vi "Audio Plugin UI Meas Ser1.vi"() -> ()   [LabVIEW 2021]
uses:
  <vilib>/PDM Acquisition Toolkit/shared/controls/i2s frame size.ctl
  <vilib>/PDM Acquisition Toolkit/host/Classes/Tasks/PDM Tasks/Controls/Acquisition Mode.ctl
  <vilib>/addons/_NISVFA/_Shared subVIs/Controls/svc_Window.ctl
  <vilib>/addons/_NISVFA/_Shared subVIs/Common/SVL Set dB Reference (1 Ch).vi
  <vilib>/addons/Sound and Vibration/svt_Level/SVL AC & DC Level (Time) (1 Ch).vi
  <vilib>/addons/_NISVFA/_Spectrum Processing/SVFA Get Spectrum Subset.vi
  <vilib>/addons/_NISVFA/_Spectrum Processing/SVFA Get Spectrum Subset (Complex) (1 Ch).vi
  <vilib>/addons/_NISVFA/_Shared subVIs/Common/svc_Window Parameters.vi
  <vilib>/addons/_NISVFA/_Shared subVIs/Common/svc_Extract Single Tone Information (complex).vi
  <vilib>/addons/_NISVFA/_Shared subVIs/Common/svc_Check Frequency Range in Spectrum.vi
  <vilib>/addons/_NISVFA/_Spectrum Processing/SVFA Unit Conversion.vi
  <vilib>/addons/_NISVFA/_Spectrum Processing/SVFA Unit Conversion (Complex) (1 Ch).vi
  <vilib>/addons/_NISVFA/_Spectrum Processing/SVFA Spectrum Peak Search.vi
  <vilib>/addons/_NISVFA/_Spectrum Processing/SVFA Spectrum Peak Search (1 Ch).vi
  <vilib>/addons/_NISVFA/_Shared subVIs/Common/svc_Spectrum Units.vi
  <vilib>/addons/_NISVFA/_Shared subVIs/Common/SVL Set dB Reference (variant).vi
  <vilib>/addons/_NISVFA/_Shared subVIs/Common/svc_Get SV Channel Info.vi
  <vilib>/Analysis/baseanly.llb/Mean.vi
  <vilib>/Analysis/baseanly.llb/Mean (DBL).vi
  <vilib>/addons/_NISVFA/_Shared subVIs/Windowing/svfa_Scaled Time Domain Window (Array).vi
  <vilib>/addons/_NISVFA/_Shared subVIs/Common/svc_Build Unit Label for Frequency Range.vi
  <vilib>/addons/_NISVFA/_Spectrum Processing/SVFA Get Tone Amplitude and Phase (1 Ch).vi
  <vilib>/addons/_NISVFA/_Spectrum Processing/subVIs/svfa_Compute Complex Spectrum for Export.vi
  <vilib>/addons/_NISVFA/_Shared subVIs/Common/svc_Check Frequency Range in Bandwidth.vi
  <vilib>/addons/_NISVFA/_Shared subVIs/Common/svc_Convert Start and Stop to Start Index and Length.vi
  <vilib>/addons/_NISVFA/_Shared subVIs/Common/svc_Log View for Spectrum (1Ch).vi
  <vilib>/addons/_NISVFA/_Spectrum Processing/SVFA Unit Conversion (1 Ch).vi
  <vilib>/addons/_NISVFA/_Shared subVIs/Common/svc_Complex Datatype Defaults.vi
  <vilib>/addons/_NISVFA/_Spectrum Processing/subVIs/svfa_Spectrum Peak Search.vi
  <vilib>/addons/_NISVFA/_Shared subVIs/Common/svc_Format Value (DBL).vi
  <vilib>/addons/_NISVFA/_Shared subVIs/Common/svc_Get Weighting Enum and Labels.vi
  <vilib>/addons/_NISVFA/_Shared subVIs/Common/svc_Engineering Units to Unit Label.vi
  <vilib>/addons/_NISVFA/_Shared subVIs/Common/svc_Surround NonAlpha String with Parentheses.vi
  <vilib>/dlg_ctls.llb/Space Constant.vi
  <vilib>/addons/_NISVFA/_Shared subVIs/Common/svc_Unit Label to Engineering Units.vi
  <vilib>/addons/_NISVFA/_Spectrum Processing/subVIs/svfa_Spectrum Info Window to windowTd Type Def.vi
  <vilib>/Analysis/4window.llb/Force Window.vi
  <vilib>/Analysis/4window.llb/Force Window (DBL).vi
  <vilib>/Analysis/4window.llb/Exponential Window.vi
  <vilib>/Analysis/4window.llb/Exponential Window (DBL).vi
  <vilib>/addons/_NISVFA/_Spectrum Processing/subVIs/svfa_Window Frequency Response.vi
  <vilib>/addons/_NISVFA/_Spectrum Processing/subVIs/svfa_Window Frequency Response (double array).vi
  <vilib>/Analysis/baseanly.llb/Dot Product.vi
  <vilib>/Analysis/baseanly.llb/Complex Dot Product.vi
  <vilib>/addons/_NISVFA/_Shared subVIs/Common/svc_Unwrap Phase.vi
  <vilib>/addons/_NISVFA/_Shared subVIs/Common/svc_Convert Spectrum Array to dB.vi
  <vilib>/addons/_NISVFA/_Spectrum Processing/subVIs/svfa_Conversion Utility (spectrum info).vi
  <vilib>/addons/_NISVFA/_Spectrum Processing/subVIs/svfa_Peak Rough Search Indices.vi
  <vilib>/addons/_NISVFA/_Shared subVIs/Common/svc_Unit Label Lexical Class.vi
  <vilib>/addons/_NISVFA/_Spectrum Processing/subVIs/svfa_Rect Window Frequency Response.vi
  <vilib>/addons/_NISVFA/_Spectrum Processing/subVIs/svfa_Cosine Window Coefficients.vi
  <vilib>/addons/_NISVFA/_Spectrum Processing/subVIs/svfa_Peak to RMS to Peak2Peak.vi
  <vilib>/addons/_NISVFA/_Spectrum Processing/subVIs/svfa_Mag to Mag2.vi
  <vilib>/addons/_NISVFA/_Spectrum Processing/subVIs/svfa_Linear to dB.vi
  <vilib>/addons/_NISVFA/_Spectrum Processing/subVIs/svfa_dBrefA to dBrefB.vi
  <vilib>/addons/_NISVFA/_Spectrum Processing/subVIs/svfa_Spectrum to Spectral Density.vi
  <vilib>/PDM Acquisition Toolkit/host/API/Public/Create Tasks/Create I2S Input Task.vi
  <vilib>/PDM Acquisition Toolkit/host/API/Public/Configure/Timing/Configure Timing - I2S Input Slave.vi
  <vilib>/PDM Acquisition Toolkit/host/API/Public/Configure/PDM Channel/Configure Microphone Sensitivity FSPA - I2S Input Task.vi
  <vilib>/PDM Acquisition Toolkit/host/API/Public/Commit/Commit I2S Input Task.vi
  <vilib>/DAQmx/create/channels.llb/DAQmx Create Channel (AO-FuncGen).vi
  <vilib>/addons/_NISVFA/_Shared subVIs/Common/svc_Caller VI Returned in Error Source.vi
  <vilib>/addons/_NISVFA/_Shared subVIs/Common/svc_Get Window Info.vi
  <vilib>/Analysis/0measdsp.llb/Scaled Time Domain Window.vi
  <vilib>/Analysis/0measdsp.llb/Scaled Time Domain Window (DBL).vi
  <vilib>/Utility/error.llb/Error Cluster From Error Code.vi
  <vilib>/Analysis/baseanly.llb/Std Deviation and Variance.vi
  <vilib>/addons/Sound and Vibration/svt_Distortion/subVIs/sv_Check Data Valid (Audio) (1 Ch).vi
  <vilib>/addons/_NISVFA/_Shared subVIs/Common/svc_Convert Frequency to Frequency String.vi
  <vilib>/Analysis/4window.llb/window parameters.vi
  <vilib>/Analysis/4window.llb/Window Properties.vi
  <vilib>/Analysis/4window.llb/Window Properties by Name.vi
  <vilib>/addons/_NISVFA/_Spectrum Processing/subVIs/svfa_Spectrum Peak Tone Search and Estimation (complex).vi
  <vilib>/measure/masignal.llb/Tones and Noise Waveform.vi
  <vilib>/addons/_NISVFA/_Shared subVIs/Common/svc_FFT with Window.vi
  <vilib>/Analysis/1siggen.llb/Square Wave.vi
  <vilib>/addons/_NISVFA/_Spectrum Processing/subVIs/svfa_Three Finger Peak Search.vi
  <vilib>/addons/Sound and Vibration/svt_Distortion/subVIs/sv_Peak View Amplitude (1 Ch).vi
  <vilib>/addons/Sound and Vibration/svt_Level/SVL AC & DC Level (Time) (N Ch).vi
  <vilib>/addons/_NISVFA/_Shared subVIs/Common/SVL Set dB Reference (N Ch - 1 Ref).vi
  <vilib>/addons/Sound and Vibration/svt_Single Tone Measurements/SVT Dynamic Range (Frequency) (1 Ch).vi
  <vilib>/addons/Sound and Vibration/svt_Distortion/SVT SNR without Harmonics (Frequency) (1 Ch).vi
  <vilib>/addons/Sound and Vibration/svt_Single Tone Measurements/SVT Gain (Time) (1 Ch).vi
  <vilib>/PDM Acquisition Toolkit/host/API/Public/Start/Start I2S Input Task.vi
  <vilib>/PDM Acquisition Toolkit/host/API/Public/Read/Read I2S Waveform.vi
  <vilib>/PDM Acquisition Toolkit/host/API/Public/Clear/Clear I2S Input Task.vi
  <vilib>/addons/Sound and Vibration/svt_Single Tone Measurements/SVT Spurious Free Dynamic Range (Frequency) (1 Ch).vi
  <vilib>/addons/Sound and Vibration/svt_Weighting/SVT Weighting Filter (N Ch).vi
  <vilib>/PDM Acquisition Toolkit/host/Classes/Tasks/PDM Tasks/PDM Task.lvclass
  <vilib>/PDM Acquisition Toolkit/host/API/PDM Acquisition Toolkit.lvlib
  <vilib>/addons/Sound and Vibration/svt_Single Tone Measurements/SoundVib_SingleTone.lvlib
  <vilib>/addons/Sound and Vibration/svt_Distortion/SoundVib_Distortion.lvlib
  <vilib>/PDM Acquisition Toolkit/shared/PDM Shared.lvlib
  <vilib>/addons/Sound and Vibration/svt_Weighting/SoundVib_ABCWeighting.lvlib
panel:
  out "MeasTable":string[][](table)
  out "MeasGraphs":enum32{"Time Domain", "Histogram", "DNL", "INL"}(tab)
  out "TimeDomain":waveform(dbl)[](graph) caption="AC"
  in  "Weighting":T1(ring) caption="WEIGHTING"
  in  "Bits per Sample":u32=24 caption="BITS PER SAMPLE"
  in  "DUT FULL SCALE (V pk)":dbl=3.16 format="%.3p"
  out "error out":errorcluster
  out "Sampling Rate":dbl=192000.0 format="%#_6p"
  in  "sample rate (S/s)":dbl=192000.0
  in  "Playback .WAV File?":bool caption="PLAYBACK .WAV FILE?"
  in  "I2S Data Latch at SCK Cycle":u8=50 caption="DATA LATCH AT SCK" format="%.0f%"
  in  "I2S Logic Level":enum16{"3.3 V", "1.8 V", "1.2 V"}(ring) caption="LOGIC LEVEL"
  in  "I2S Frame Size":enum16{"32bits", "64bits"}(ring) caption="FRAME SIZE"
  in  "I2S Number of Words":u32=19200 caption="NO OF WORDS"
  in  "I2S Word Length":u32=24 caption="WORD LENGTH"
  in  "I2S Clock Rate":u32=12288000 caption="CLOCK RATE" format="%#.6pHz"
  in  "THD Maximum Harmonic":u32=9 caption="MAX HARMONIC"
  in  "Measurement Band Stop":dbl=20000.0 caption="BAND STOP" format="%#_6pHz"
  in  "Measurement Band Start":dbl=20.0 caption="BAND START" format="%#_6pHz"
  in  "DSG amplitude":dbl=1.0 caption="AMPLITUDE" format="%#_6pV"
  in  "DSG frequency":dbl=1000.0 caption="FREQUENCY" format="%#_6pHz"
  in  "DSG resource name":string="4468/ao0" caption="RESOURCE NAME"
  in  "Mic sensitivity (FS/Pa)":dbl=0.34762 caption="MIC SENSITIVITY" format="%.3fFS/Pa"
  in  "I2S Channel List":string="PXI1Slot7\\I2Si 0" caption="CHANNEL LIST"
  in  "Playback .WAV file path":path caption="PLAYBACK .WAV FILE PATH"
  in  "Record .WAV File?":bool caption="RECORD .WAV FILE?"
  in  "Record wave file path":path caption="RECORD .WAV FILE PATH"
  # "Analog Source"
  # "I2S Setting"
  # "Measurement"
  # "Record"
  # "Playback"
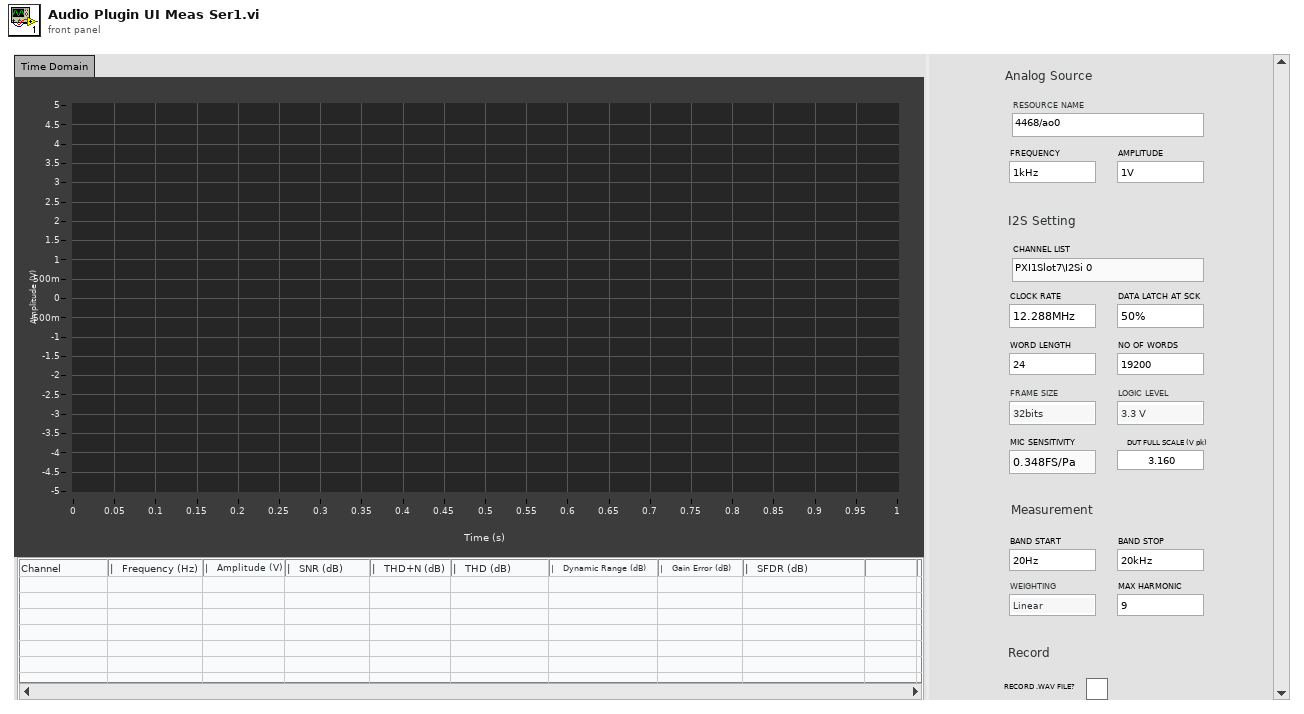
[diagram p1: front panel]
types:
  T1 = enum16{"Linear", "A-Weighting", "B-Weighting", "C-Weighting"}
  T2 = cluster{"band start (Hz)":dbl, "band stop (Hz)":dbl}
  T3 = typedef "PDM Shared.lvlib/i2s frame size.ctl" = enum16{"32bits", "64bits"}
  T4 = cluster{"frequency range":cluster{"band start (Hz)":dbl, "band stop (Hz)":dbl}, "THD maximum harmonic":i32, "amplitude":dbl, "frequency (Hz)":dbl, "output channel":tag, "microphone sensitivity (FS/Pa)":dbl, "number of words":i32, "channel list":string, "logic level":enum16{"3.3 V", "1.8 V", "1.2 V"}, "I2S serial clock rate 2":u32, "frame size":T3, "word length":u32, "Data Latch at SCK cycle":u8, "Playback .WAV File?":bool, "Record .WAV File?":bool, "Record wave file path":path, "Playback .WAV file path":path, "number of channels":i32, "DUT full scale (V pk)":dbl, "weighting":u16}
  T5 = typedef "PDM Acquisition Class Library.lvlib/PDM Task.lvclass/Acquisition Mode.ctl" = enum16{"Finite", "Continuous"}
  T6 = cluster{"SNR units":enum16{"dB", "linear ratio", "%"}, "detected fundamental amplitude units":enum16{"EU rms", "EU peak", "EU peak-peak"}}
  T7 = cluster{"gain units":enum16{"dB", "linear ratio"}, "detected fundamental amplitude units":enum16{"EU rms", "EU peak", "EU peak-peak"}}
  T8 = typedef "PDM Acquisition Class Library.lvlib/I2S Input Task.lvclass/DVR I2S Input Task.ctl" = refnum<data-value>
  T9 = typedef "svc_Window.ctl" = u32
  T10 = typedef "svc_Spectrum Info.ctl" = cluster{"channel name":string, "description":string, "x-axis units":T11, "spectral info":cluster{"spectrum type":T12, "linear/dB":enum16{"linear", "dB"}, "window":u16, "window size":i32, "FFT size":i32}, "engineering units":T13, "custom label":string, "dB reference [EU]":dbl, "peak units":enum16{"rms", "peak", "peak-peak"}, "weighting filter":T14, "spectral density?":bool, "unit label":string, "spectrum skewed?":bool, "complimentary spectrum units":T15}
  T11 = typedef "svc_X-Axis Units.ctl" = u16
  T12 = typedef "svc_Spectrum Type.ctl" = enum16{"FFT Spectrum [complex]", "Amplitude [Magnitude]", "Power [Magnitude^2]", "Cross Spectrum [complex]", "Frequency Response [Complex]"}
  T13 = typedef "svc_Engineering Units Text Ring.ctl" = u16
  T14 = typedef "svc_Weighting Filter Text Ring.ctl" = u16
  T15 = typedef "svc_Complimentary Spectrum Units.ctl" = enum16{"none", "radians", "degrees", "cycles", "imaginary"}
  T16 = cluster{"complex spectrum response":cluster{"f0":dbl, "df":dbl, "complex spectrum":cdb[]}, "spectrum info":T10}
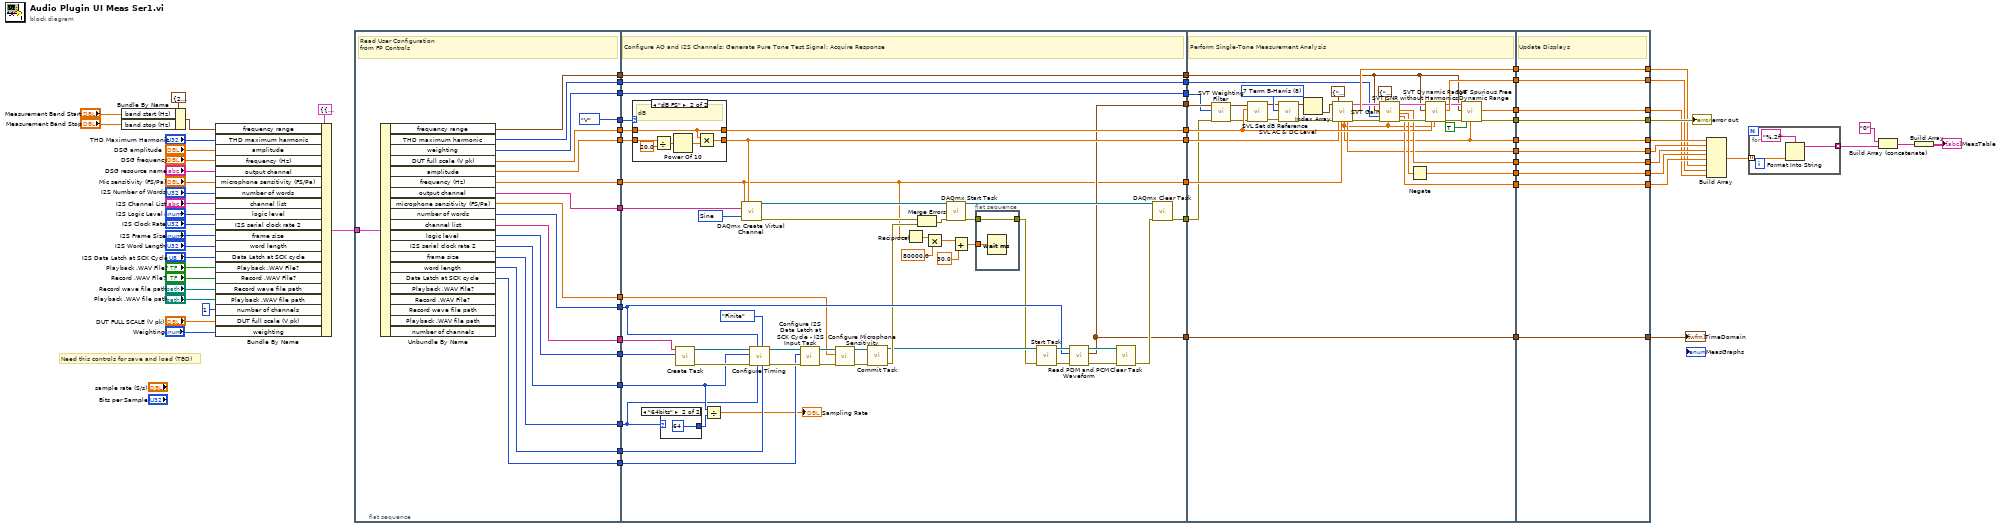
[diagram p0: block diagram]
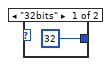
[diagram p2: hidden frame]
diagram:
  # "Need this controls for save and load (TBD)"
  n1 = Bundle By Name(cluster=T2 {"band start (Hz)"=20.0, "band stop (Hz)"=20000.0} ("frequency range"), "band start (Hz)"="Measurement Band Start", "band stop (Hz)"="Measurement Band Stop") -> (w41:T2)
  n2 = Bundle By Name(cluster=T4 {"frequency range"={"band start (Hz)"=20.0, "band stop (Hz)"=20000.0}, "THD maximum harmonic"=9, "amplitude"=1.0, "frequency (Hz)"=1000.0, "output channel"="Dev1/ao0", "microphone sensitivity (FS/Pa)"=0.34762, "number of words"=19200, "channel list"="PXI1Slot7\\I2Si 0", "logic level"=enum."3.3 V", "I2S serial clock rate 2"=12288000, "frame size"=enum."64bits", "word length"=24, "Data Latch at SCK cycle"=50, "Playback .WAV File?"=FALSE, "Record .WAV File?"=FALSE, "Record wave file path"=path "", "Playback .WAV file path"=path "", "number of channels"=1, "DUT full scale (V pk)"=3.16, "weighting"=0}, "frequency range"=w41, "THD maximum harmonic"="THD Maximum Harmonic", "amplitude"="DSG amplitude", "frequency (Hz)"="DSG frequency", "output channel"="DSG resource name", "microphone sensitivity (FS/Pa)"="Mic sensitivity (FS/Pa)", "number of words"="I2S Number of Words", "channel list"="I2S Channel List", "logic level"="I2S Logic Level", "I2S serial clock rate 2"="I2S Clock Rate", "frame size"="I2S Frame Size", "word length"="I2S Word Length", "Data Latch at SCK cycle"="I2S Data Latch at SCK Cycle", "Playback .WAV File?"="Playback .WAV File?", "Record .WAV File?"="Record .WAV File?", "Record wave file path"="Record wave file path", "Playback .WAV file path"="Playback .WAV file path", "number of channels"=1, "DUT full scale (V pk)"="DUT FULL SCALE (V pk)", "weighting"="Weighting") -> (w23:T4)
  n3 = flat-sequence {
    tunnel: [w89] -> w75
    tunnel: [w86] -> w74
    tunnel: [w85] -> w73
    tunnel: [w88] -> w72
    tunnel: [w87] -> w71
    tunnel: [enum16{"V", "dB FS"}."V" ("amplitude units")] -> w70
    tunnel: [w80] -> w69
    tunnel: [w81] -> w68
    tunnel: [w77] -> w67
    tunnel: [w83] -> w66
    tunnel: [w78] -> w65
    tunnel: [w79] -> w64
    tunnel: [w82] -> w63
    tunnel: [w84] -> w47
    tunnel: w23 -> [w91]
    tunnel: [w90] -> w22
    tunnel: [w76] -> w3
    tunnel: w75 -> [w138]
    tunnel: w74 -> [w98]
    tunnel: w73 -> [w136]
    tunnel: w72 -> [w141]
    tunnel: w71 -> [w140]
    tunnel: w70 -> [w137]
    tunnel: [w142] -> w62
    tunnel: [w139] -> w61
    tunnel: [w138] -> w60
    tunnel: [w135] -> w59
    tunnel: [w98] -> w58
    tunnel: [w106] -> w57
    tunnel: [w130] -> w56
    tunnel: w69 -> [w117]
    tunnel: w68 -> [w116]
    tunnel: w67 -> [w115]
    tunnel: w66 -> [w114]
    tunnel: w65 -> [w113]
    tunnel: w64 -> [w112]
    tunnel: w63 -> [w111]
    tunnel: w47 -> [w108]
    tunnel: w22 -> [w142]
    tunnel: [w106] -> w18
    tunnel: w3 -> [w105]
    tunnel: [w105] -> w2
    tunnel: [w178] -> w55
    tunnel: [w177] -> w54
    tunnel: [w164] -> w53
    tunnel: [w176] -> w52
    tunnel: [w175] -> w51
    tunnel: [w174] -> w50
    tunnel: [w173] -> w49
    tunnel: [w163] -> w48
    tunnel: w62 -> [w162]
    tunnel: w61 -> [w180]
    tunnel: w60 -> [w170]
    tunnel: w59 -> [w179]
    tunnel: w58 -> [w172]
    tunnel: w57 -> [w159]
    tunnel: w56 -> [w156]
    tunnel: [w167] -> w19
    tunnel: w18 -> [w167]
    tunnel: [w160] -> w17
    tunnel: w2 -> [w155]
    tunnel: w55 -> [w193]
    tunnel: w54 -> [w192]
    tunnel: w53 -> [w200]
    tunnel: w52 -> [w194]
    tunnel: w51 -> [w195]
    tunnel: w50 -> [w196]
    tunnel: w49 -> [w197]
    tunnel: w48 -> [w198]
    tunnel: [w200] -> w46
    tunnel: [w199] -> w20
    tunnel: w19 -> [w199]
    tunnel: w17 -> [w191]
    tunnel: [w198] -> w16
    tunnel: [w197] -> w15
    tunnel: [w196] -> w14
    tunnel: [w195] -> w13
    tunnel: [w194] -> w12
    tunnel: [w193] -> w11
    tunnel: [w192] -> w10
    tunnel: [w191] -> w9
    frame #0 {
      # "Read User Configuration\nfrom FP Controls"
      n4 = Unbundle By Name(w91) -> ("frequency range"=w90:T2, "THD maximum harmonic"=w89:i32, "weighting"=w76:u16, "DUT full scale (V pk)"=w88:dbl, "amplitude"=w87:dbl, "frequency (Hz)"=w86:dbl, "output channel"=w85:tag, "microphone sensitivity (FS/Pa)"=w84:dbl, "number of words"=w83:i32, "channel list"=w82:string, "logic level"=w81:enum16{"3.3 V", "1.8 V", "1.2 V"}, "I2S serial clock rate 2"=w80:u32, "frame size"=w79:T3, "word length"=w78:u32, "Data Latch at SCK cycle"=w77:u8)  [unwired: 5 out]
    }
    frame #1 {
      w107 = 14751 items=["Sine"=14751, "Triangle"=14752, "Square"=14753, "Sawtooth"=14754] ("type")
      # "Configure AO and I2S Channels; Generate Pure Tone Test Signal; Acquire Response"
      n5 = case shown="\"dB FS\"" w137 {
        tunnel: [w148 w150] -> w135
        tunnel: w140 -> [w148 w154]
        tunnel: w141 -> [w147 w149]
        tunnel: [w147 w149] -> w139
        frame Default {
          # "V"
        }
        frame "dB FS" {
          # "dB"
          n6 = Divide(x=w154, y=20.0) -> (x/y=w152:dbl)
          n7 = Power Of 10(x=w152) -> (10^x=w151:dbl)
          n8 = Multiply(x=w149, y=w151) -> (x*y=w150:dbl)
        }
      }
      n9 = case shown="\"64bits\"" w112 {
        tunnel: [u8 32 ("frame size") u8 64 ("frame size")] -> w118
        frame "32bits" {
        }
        frame "64bits" {
        }
      }
      n10 = call-poly <vilib>:"Create Task.vi"("logic level"=w116, "channel list"=w111) -> ("error out"=w124:errorcluster, "I2S input task out"=w123:T8)  [unwired: 8 in]
      n11 = Divide(x=w117, y=w118) -> (x/y=→"Sampling Rate":dbl)
      n12 = call-poly <vilib>:"DAQmx Create Virtual Channel.vi"("frequency"=w98, "amplitude"=w135, "physical channels"=w136, "type"=w107) -> ("task out"=w132:refnum<k21>, "error out"=w134:errorcluster)  [unwired: 10 in]
      n13 = call-poly <vilib>:"Configure Timing.vi"("word length"=w113, "acquisition mode"=Acquisition_Mode."Finite", "frame size"=w112, "number of words"=w114, "error in"=w124, "I2S serial clock rate"=w117, "I2S input task in"=w123) -> ("error out"=w122:errorcluster, "I2S input task out"=w119:T8)  [unwired: 3 in]
      n14 = call <vilib>:"Configure I2S Data Latch at SCK Cycle - I2S Input Task.vi"("error in"=w122, "data latch at SCK cycle"=w115, "I2S input task in"=w119) -> ("error out"=w121:errorcluster, "I2S input task out"=w120:T8)  [unwired: 7 in]
      n15 = call-poly <vilib>:"Configure Microphone Sensitivity.vi"("error in"=w121, "microphone sensitivity (FS/Pa)"=w108, "I2S input task in"=w120) -> ("error out"=w104:errorcluster, "I2S input task out"=w103:T8)  [unwired: 7 in]
      n16 = call-poly <vilib>:"Commit Task.vi"("error in"=w104, "I2S input task in"=w103) -> ("error out"=w102:errorcluster, "I2S input task out"=w101:T8)  [unwired: 8 in]
      n17 = Reciprocal(x=w98) -> (1/x=w97:dbl)
      n18 = Merge Errors(w134, w102) -> (w133:errorcluster)
      n19 = Multiply(x=w97, y=80000.0) -> (x*y=w95:dbl)
      n20 = call <vilib>:"DAQmx Start Task.vi"("task/channels in"=w132, "error in"=w133) -> ("task out"=w131:refnum<k21>, "error out"=w99:errorcluster)  [unwired: 12 in]
      n21 = Add(x=w95, y=30.0) -> (x+y=w93:dbl)
      n22 = flat-sequence {
        tunnel: [w144] -> w100
        tunnel: w99 -> [w144]
        tunnel: w93 -> [w143]
        frame #0 {
          n23 = Wait (ms)(milliseconds to wait=w143) -> ()  [unwired: 1 out]
        }
      }
      n24 = call-poly <vilib>:"Start Task.vi"("error in"=w100, "I2S input task in"=w101) -> ("error out"=w128:errorcluster, "I2S input task out"=w127:T8)  [unwired: 8 in]
      n25 = call-poly <vilib>:"Read PDM and PCM Waveform.vi"("error in"=w128, "words per channel"=w114, "I2S input task in"=w127) -> ("error out"=w126:errorcluster, "I2S waveforms"=w106:waveform(dbl)[], "I2S input task out"=w125:T8)  [unwired: 4 in, 2 out]
      n26 = call-poly <vilib>:"Clear Task.vi"("error in"=w126, "I2S input task in"=w125) -> ("error out"=w110:errorcluster)  [unwired: 9 in]
      n27 = call <vilib>:"DAQmx Clear Task.vi"("task in"=w131, "error in"=w110) -> ("error out"=w130:errorcluster)  [unwired: 13 in]
    }
    frame #2 {
      w189 = T9 8 items=["None"=0, "Hanning"=1, "Hamming"=2, "Blackman-Harris"=3, "Exact Blackman"=4, "Blackman"=5, "Flat Top"=6, "4 Term B-Harris "=7, "7 Term B-Harris"=8, "Low Sidelobe"=9, "Force"=64, "Exponential"=65, "Blackman Nuttall"=11, "Triangle"=30, "Bartlett-Hanning"=31, "Bohman"=32, "Parzen"=33, "Welch"=34, "Kaiser"=60, "Dolph-Chebyshev"=61, "Gaussian"=62] ("window")
      # "Perform Single-Tone Measurement Analysis"
      n28 = call-poly <vilib>:"SVT Weighting Filter.vi"("error in (no error)"=w156, "weighting"=w155, "scaled signals [EU]"=w159) -> ("error out"=w157:errorcluster, "weighted signals [EU]"=w158:waveform(dbl)[])  [unwired: 6 in]
      n29 = call-poly <vilib>:"SVL Set dB Reference.vi"("error in (no error)"=w157, "dB reference [EU]"=w180, "scaled signals in [EU]"=w158) -> ("error out"=w188:errorcluster, "scaled signals out [EU]"=w186:waveform(dbl)[])  [unwired: 7 in]
      n30 = call-poly <vilib>:"SVL AC & DC Level.vi"("scaled signals in [EU]"=w186, "window"=w189, "error in (no error)"=w188) -> ("AC signals [EU]"=w187:waveform(dbl)[], "error out"=w168:errorcluster)  [unwired: 11 in, 4 out]
      n31 = Index Array(array=w187) -> (element=w169:waveform(dbl))  [unwired: 1 in]
      n32 = call-poly <vilib>:"SVT Gain.vi"("scaled signal [EU]"=w169, "error in (no error)"=w168, "desired units"=T7 {"gain units"=enum."dB", "detected fundamental amplitude units"=enum."EU peak"}, "amplitude [EU peak]"=w179, "expected fundamental frequency [Hz]"=w172) -> ("detected fundamental\nfrequency [Hz]"=w163:dbl, "detected fundamental\namplitude"=w173:dbl, "complex spectrum"=w171:T16, "gain"=w178:dbl, "error out"=w190:errorcluster)  [unwired: 9 in, 1 out]
      n33 = call-poly <vilib>:"SVT SNR without Harmonics.vi"("complex spectrum"=w171, "frequency range"=w162, "maximum harmonic"=w170, "error in (no error)"=w190, "desired units"=T6 {"SNR units"=enum."dB", "detected fundamental amplitude units"=enum."EU rms"}, "expected fundamental frequency [Hz]"=w163) -> ("complex spectrum"=w184:T16, "SNR (without harmonics)"=w174:dbl, "SINAD"=w183:dbl, "THD"=w176:dbl, "error out"=w185:errorcluster)  [unwired: 6 in, 3 out]
      n34 = Negate(x=w183) -> (-x=w175:dbl)
      n35 = call-poly <vilib>:"SVT Dynamic Range.vi"("complex spectrum"=w184, "frequency range"=w162, "error in (no error)"=w185, "full scale amplitude [EU peak]"=w180, "expected fundamental\nfrequency [Hz]"=w163) -> ("dup complex spectrum"=w166:T16, "dynamic range"=w177:dbl, "error out"=w165:errorcluster)  [unwired: 9 in, 3 out]
      n36 = call-poly <vilib>:"SVT Spurious Free Dynamic Range.vi"("complex spectrum"=w166, "frequency range"=w162, "error in (no error)"=w165, "exclude harmonics"=TRUE, "expected fundamental\nfrequency [Hz]"=w163) -> ("spurious free dynamic range"=w160:dbl, "error out"=w164:errorcluster)  [unwired: 7 in, 6 out]
    }
    frame #3 {
      # "Update Displays"
    }
  }
  n37 = Build Array(w16, w15, w14, w13, w12, w11, w10, w9) -> (w8:dbl[])
  n38 = for {
    tunnel: w8 -> [w203] mode=indexing
    tunnel: [w201] -> w6 mode=indexing
    n39 = Format Into String(format string="%.2f", w203) -> (resulting string=w201:string)  [unwired: 2 in, 1 out]
  }
  n40 = Build Array (concatenate)("0", w6) -> (w5:string[])
  n41 = Build Array(w5) -> (→"MeasTable":string[][])
  "error out" <- w46
  "TimeDomain" <- w20
